vi "cRIO-9076_RT.vi"() -> ()   [LabVIEW 2012]
doc: "This VI shows an example of how to implement a closed loop position move using the NI 9505. The position loop is implemented using PID. The output of the loop is used as the command for the current loop, which then sets the PWM duty cycle for the motor. This example assumes that an encoder is connected for position and velocity feedback. This example does not implement advanced motion features such as trajectory generation and splining."
uses:
  <vilib>/LabVIEW Targets/FPGA/cRIO/cRIO-9505/controls.llb/_nicrio_cRIO-9505_DriveStatus.ctl
  <vilib>/Platform/TimedLoop/XDataNode/timing_clust.ctl
  <vilib>/Platform/TimedLoop/XDataNode/nitl_modes.ctl
  <vilib>/Platform/TimedLoop/XDataNode/wakeup.ctl
  <vilib>/FPGAPlugInAG/cRIO-9076/niLvFpga_Open_cRIO-9076.vi
  <vilib>/Utility/error.llb/Error Cluster From Error Code.vi
  <vilib>/rvi/errors/niLvFpgaAdjustHostInterfaceError.vi
  <vilib>/Analysis/3filter.llb/Zero Phase Filter (DBL).vi
  <vilib>/FPGAPlugInAG/cRIO-9076/niLvFpga_Close_cRIO-9076.vi
  <vilib>/rvi/interface/nirviOpenFPGA/nirviOpenFPGA.xnode
  FPGA Bitfiles/GWiz32_FPGATarget2_PositionControl(_zhcafk1Bo4c.lvbitx
  C:/Temp/National Instruments Downloads/LabVIEW FPGA English/2012SP1/cRIO-9076_FPGA.vi
  <vilib>/rvi/interface/nirviReadWriteControl/nirviReadWriteControl.xnode
  <vilib>/Platform/TimedLoop/XDataNode/XDataNode.xnode
  <vilib>/rvi/interface/nirviCloseFPGA/nirviCloseFPGA.xnode
  NiFpgaLv.dll
  <vilib>/Analysis/NI_AALPro.lvlib
  <vilib>/Platform/TimedLoop/XDataNode/XDNodeRunTimeDep.lvlib
  <vilib>/Analysis/NI_AALBase.lvlib
panel:
  in  "Tab Control":enum32{"Controls", "Plot_data"}(tab)
  in  "samples":i32=10000
  in  "signal type":T1(ring)=enum."square"
  in  "cycles":dbl=1.0 format="%0.2f"
  in  "delay":dbl=180.0 format="%0.2f"
  out "Ball Position (V)":dbl(slide) min=-0.2 max=0.2 step=0.001 scale=0.0..12.0 scale format="%.1f"
  out "Gear Angle Theta (V)":dbl(knob) scale=0.0..12.0 scale format="%.2f"
  in  "MANUAL\n/AUTO":bool caption="Auto"
  in  "Motor Voltage 2":dbl(slide) min=-5.0 max=5.0 step=0.01 scale=-6.0..6.0
  out "Motor Voltage":dbl(knob) scale=-6.0..6.0 scale format="%.1f"
  in  "Stiction V \nOffset cw":dbl step=0.01 format="%.4f"
  in  "dc offset":dbl=0.195 format="%.3f"
  in  "amplitude":dbl=0.075 format="%.3f"
  in  "Period(ms)":dbl=50.0 min=0.1 max=1000.0 format="%.2f"
  out "Period OK":bool=TRUE
  in  "STOP":bool
  out "Missed":i16
  in  "Path":path=path "cRIO-9076_RT.vi"
  in  "Stiction V \nOffset ccw":dbl step=0.01 format="%.4f"
  out "RT Plot":cluster{dbl, "ServoAng":dbl, "BallPosn":dbl}(graph)={0.0, "ServoAng"=7.103515625, "BallPosn"=10.50048828125}
  in  "Data plot":bool
  in  "Ball filter":bool=TRUE
  in  "Gear filter":bool=TRUE
  out "Graph":T2(graph)
  out "error out":errorcluster
  # "GWiz v3.2"
  # "Ball & Beam"
  # "Reference\nGenerator"
  # "F2017 2011"
  # "Press Ctrl-H for help"
  # "Export data: right click plot"
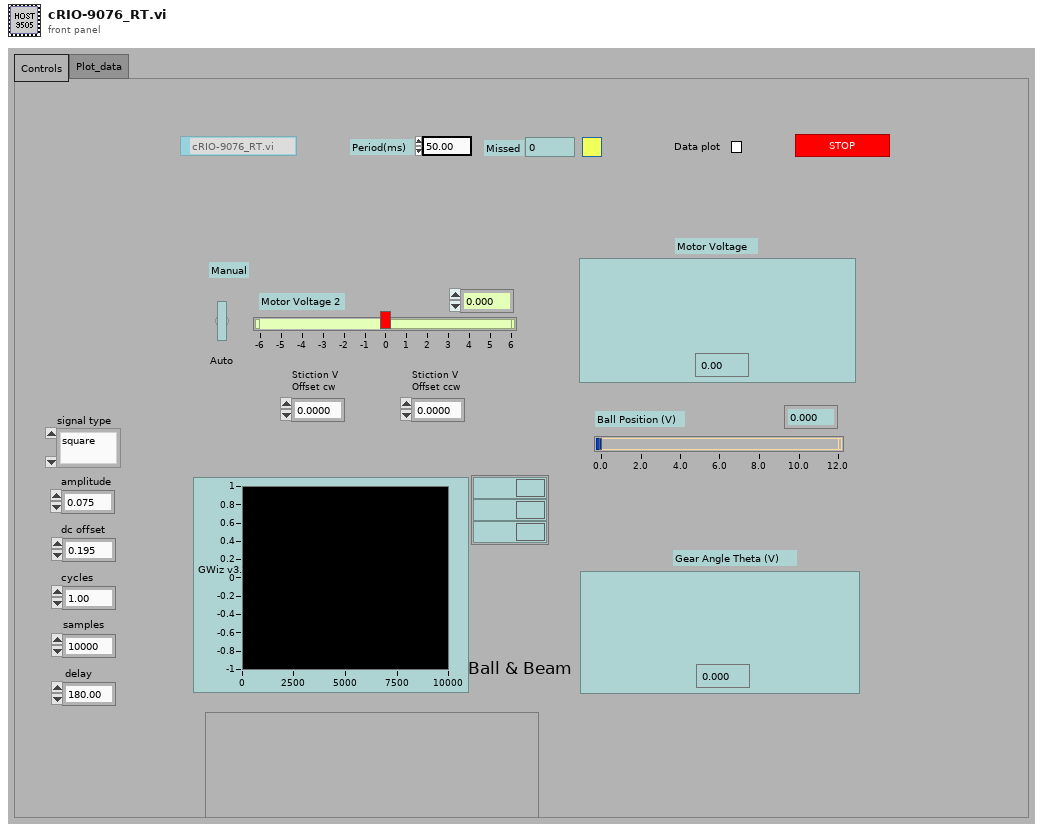
[diagram p1: front panel]
types:
  T1 = enum16{"sine", "cosine", "triangle", "square", "sawtooth", "increasing ramp", "decreasing ramp"}
  T2 = cluster{"Initial time":dbl, dbl, "Data to Plot":dbl[][]}
  T3 = typedef "_nicrio_cRIO-9505_DriveStatus.ctl" = enum8{"Enabled", "Disabled", "Disabled by Drive Fault", "Disabled by Temp. Fault", "Disabled by E-Stop", "Unknown"}
  T4 = typedef "XDNodeRunTimeDep.lvlib/timing_clust.ctl" = cluster{"Expected End [f-1]":u64, "Actual End [f-1]":u64, "Finished Late? [f-1]":bool, "Expected End [i-1]":u64, "Actual End [i-1]":u64, "Finished Late? [i-1]":bool, "Expected Start [i]":u64, "Actual Start [i]":u64, "Expected Start [f]":u64, "Actual Start [f]":u64, "Source Name":string, "Structure Name":string, "Period":i64, "Deadline":i64, "Offset":i64, "Start":i64, "Priority":i32, "Timeout":i32, "Mode":T5, "Wakeup Reason":T6, "Error":errorcluster, "Source Type":string, "Secondary Source Type":string, "Global End Time":u64, "Global Start Time":u64, "Frame Duration":u64, "Iteration Duration":u64, "Assigned CPU":i32, "I/O Scan Engine Mode":u32}
  T5 = typedef "XDNodeRunTimeDep.lvlib/nitl_modes.ctl" = enum32{"No Change", "Process missed periods, maintain original phase", "Discard missed periods, maintain original phase", "Process missed periods, ignore original phase", "Discard missed periods, ignore original phase"}
  T6 = typedef "XDNodeRunTimeDep.lvlib/wakeup.ctl" = enum32{"Normal", "Aborted", "Asynchronous wakeup", "Timing source error", "Timed loop error", "Timeout"}
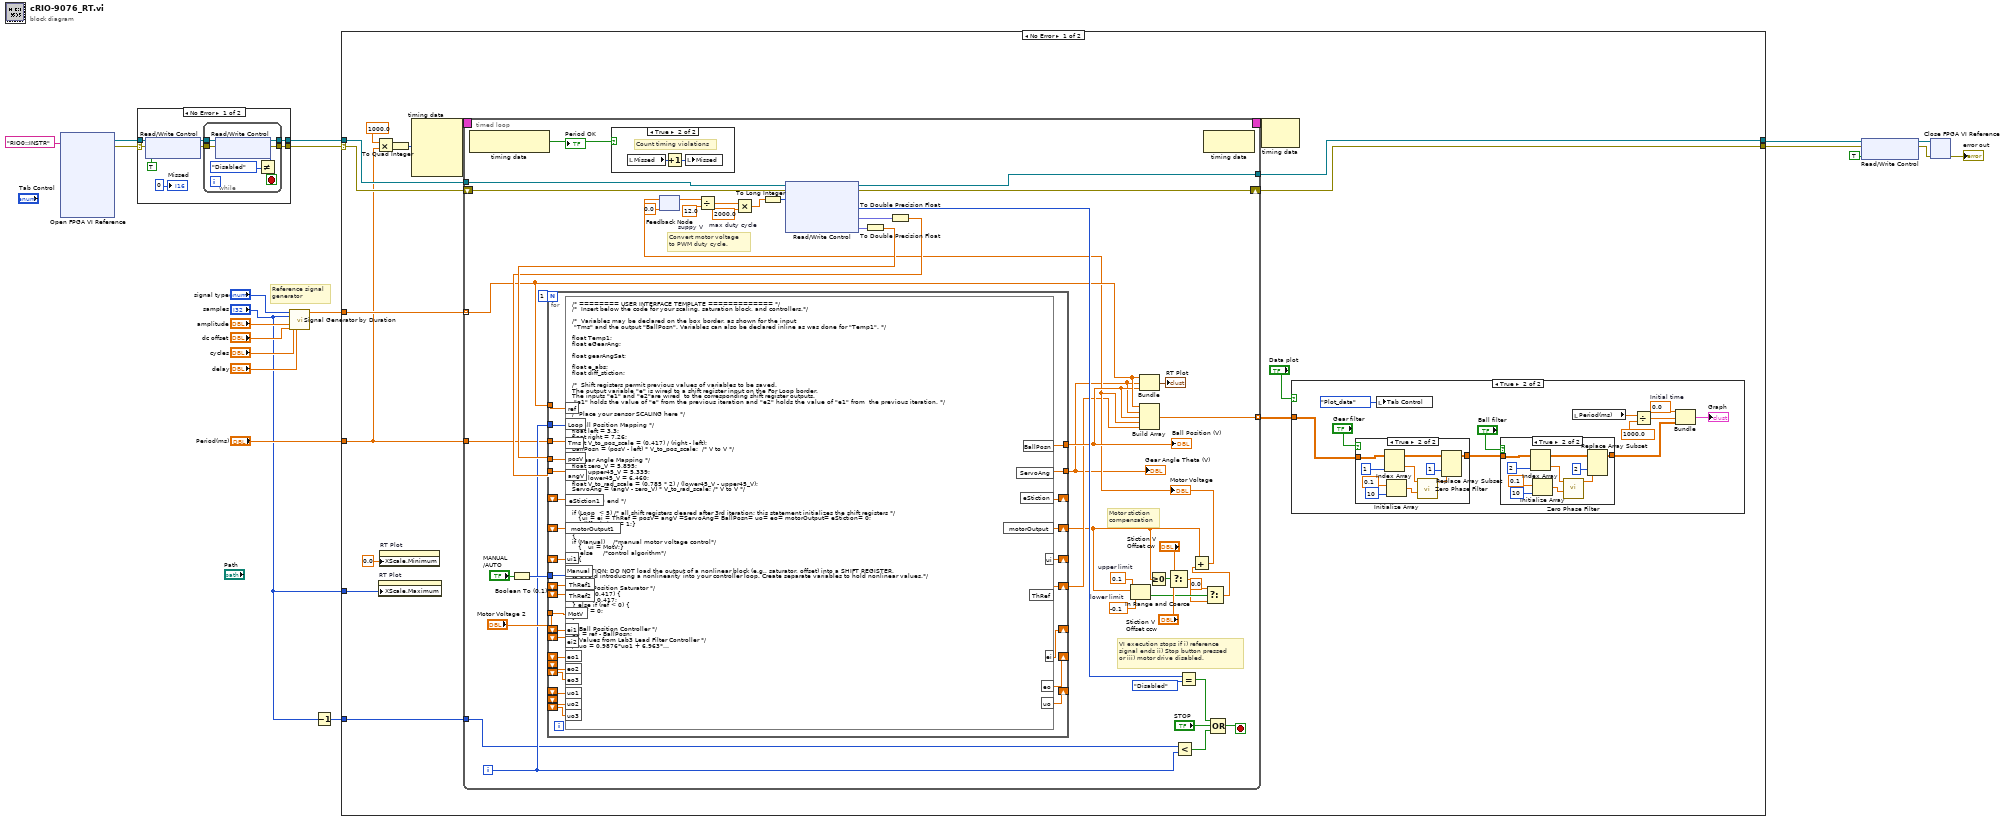
[diagram p0: block diagram]
diagram:
  # "Reference signal\ngenerator"
  n1 = xnode "Open FPGA VI Reference"("resource name"="RIO0::INSTR") -> ("FPGA VI Reference Out"=w7:refnum<k20>, "error out"=w14:errorcluster)  [unwired: 1 in]
  n2 = case shown="No Error" w14 {
    selector: w14 -> [w23 w36]
    tunnel: w7 -> [w26 w37]
    tunnel: [w28 w37] -> w15
    tunnel: [w22 w36] -> w13
    frame No Error {
      n3 = xnode "Read/Write Control"("FPGA VI Reference In"=w26, "error in"=w23, "Enable Drive"=TRUE) -> ("FPGA VI Reference Out"=w25:refnum<k20>, "error out"=w24:errorcluster)
      n4 = while {
        tunnel: [w35] -> w28
        tunnel: w25 -> [w31]
        tunnel: w24 -> [w32]
        tunnel: [w29] -> w22
        stop <- w30 stop-if-true
        n5 = xnode "Read/Write Control"("FPGA VI Reference In"=w31, "error in"=w32) -> ("FPGA VI Reference Out"=w35:refnum<k20>, "error out"=w29:errorcluster, "Drive Status"=w34:T3)
        n6 = Not Equal?(x=w34, y=_nicrio_cRIO-9505_DriveStatus."Disabled") -> (x != y?=w30:bool)
      }
      "Missed" <- i16 0 ("Missed")
    }
    frame Error {
      # "Error occurred. Do not run."
    }
  }
  n7 = call <vilib>:"Signal Generator by Duration.vi"("signal type"="signal type", "# of samples"="samples", "frequency"="cycles", "amplitude"="amplitude", "dc offset"="dc offset", "phase in"="delay") -> ("signal"=w9:dbl[])  [unwired: 6 in, 3 out]
  n8 = Decrement(x="samples") -> (x-1=w2:i32)
  n9 = case shown="No Error" w13 {
    selector: w13 -> [w51 w169]
    tunnel: w15 -> [w53 w170]
    tunnel: [w42 w170] -> w20
    tunnel: [w52 w169] -> w19
    tunnel: w9 -> [w50 _]
    tunnel: w2 -> [w49 _]
    tunnel: "Period(ms)" -> [w46 _]
    tunnel: "samples" -> [w38 _]
    frame No Error {
      n10 = Multiply(x=1000.0, y=w46) -> (x*y=w44:dbl)
      n11 = property on="RT Plot" class="WFChart (strict)"("XScale.Maximum"=w38) -> ()  [unwired: 2 in, 2 out]
      n12 = property on="RT Plot" class="WFChart (strict)"("XScale.Minimum"=0.0 ("X Scale.Range:Minimum")) -> ()  [unwired: 2 in, 2 out]
      n13 = To Quad Integer(1:w44) -> (0:w43:i64)
      n14 = node-c288(w43) -> (w48:T4)  [unwired: 3 in]
      n15 = timed-loop {
        tunnel: w53 -> [w130]
        tunnel: [w128] -> w42
        shift-right: [w127] -> w52
        shift-left: w51 -> [w129]
        tunnel: w50 -> [w101] mode=indexing
        tunnel: w49 -> [w103]
        tunnel: w46 -> [w96]
        timing: w48 -> [_]
        timing-out: [_] -> w47
        tunnel: [w97] -> w41 mode=indexing
        i -> [w104]
        stop <- w124 stop-if-true
        w89 = -0.1  # lower limit
        w90 = 0.1  # upper limit
        w109 = 2000.0  # max duty cycle
        w108 = 12.0  # suppy V
        # "Convert motor voltage\nto PWM duty cycle."
        # "VI execution stops if i) reference\nsignal ends ii) Stop button pressed\nor iii) motor drive disabled."
        # "Motor stiction\ncompensation"
        n16 = node-c288() -> (w111:bool)  [unwired: 1 in]
        "Period OK" <- w111
        n17 = Boolean To (0,1)(Boolean="MANUAL\n/AUTO") -> (0, 1=w116:i16)
        n18 = case shown="True" w111 {
          frame False {
          }
          frame True {
            # "Count timing violations"
            n19 = local read "Missed"() -> (w132:i16)
            n20 = Increment(x=w132) -> (x+1=w131:i16)
            n21 = local write "Missed"(w131) -> ()
          }
        }
        n22 = feedback #1(0.0) -> (w106:dbl)
        n23 = Divide(x=w106, y=w108) -> (x/y=w107:dbl)
        n24 = Multiply(x=w107, y=w109) -> (x*y=w105:dbl)
        n25 = To Long Integer(number=w105) -> (32bit integer=w102:i32)
        n26 = xnode "Read/Write Control"("FPGA VI Reference In"=w130, "error in"=w129, "Position Setpoint"=w102) -> ("FPGA VI Reference Out"=w128:refnum<k20>, "error out"=w127:errorcluster, "Drive Status"=w126:T3, "Gear Pot"=w122:fxp<+/-,16,5>, "Ball Pot"=w121:fxp<+/-,16,5>)
        n27 = To Double Precision Float(number=w121) -> (double precision float=w119:dbl)
        n28 = To Double Precision Float(number=w122) -> (double precision float=w114:dbl)
        n29 = for {
          N: 1 -> [_]
          tunnel: w101 -> [w164]
          tunnel: w119 -> [w163]
          shift-right: [w149] -> w88
          shift-left: _ -> [w162]
          shift-right: [w161] -> _
          shift-left: _ -> [w160]
          tunnel: [w159] -> w100
          tunnel: w96 -> [w158]
          tunnel: w114 -> [w157]
          tunnel: [w156] -> w95
          tunnel: w116 -> [w155]
          tunnel: "Motor Voltage 2" -> [w154]
          shift-right: [w153] -> w98
          shift-left: _ -> [w152]
          shift-left: _ -> [w151]
          tunnel: w104 -> [w150]
          shift-left: _ -> [w148]
          shift-right: [w146] -> _
          shift-left: _ -> [w147]
          shift-left: _ -> [w145]
          shift-right: [w144] -> _
          shift-left: _ -> [w143]
          shift-left: _ -> [w142]
          shift-right: [w141] -> _
          shift-left: _ -> [w140]
          shift-right: [w139] -> _
          shift-left: _ -> [w138]
          shift-left: _ -> [w137]
          shift-left: _ -> [w136]
          n30 = formula code="/* ======== USER INTERFACE TEMPLATE ============= */\n/*  Insert below the code for your scaling, saturation block, and controllers.*/\n\n/*  Variables may be declared on the box border, as shown for the input \n \"Tms\" and the output \"BallPosn\". Variables can also be declared inline as was done for \"Temp1\". */\n\nfloat Temp1; \nfloat eGearAng;\n\nfloat gearAngSat;\n\nfloat e_abs;\nfloat diff_stiction;\n\n/*  Shift registers permit previous values of variables to be saved. \nThe output variable \"e\" is wired to a shift register input on the For Loop border.  \nThe inputs \"e1\" and \"e2\"are wired  to the corresponding shift register outputs.\n \"e1\" holds the value of \"e\" from the previous iteration and \"e2\" holds the value of \"e1\" from  the previous iteration. */\n\n/* Place your sensor SCALING here */\n\n/* Ball Position Mapping */\nfloat left = 3.3;\nfloat right = 7.26;\nfloat V_to_pos_scale = (0.417) / (right - left);\nBallPosn = (posV - left) * V_to_pos_scale;  /* V to V */\n\n/* Gear Angle Mapping */\nfloat zero_V = 5.895;\nfloat upper45_V = 5.339;\nfloat lower45_V = 6.460;\nfloat V_to_rad_scale = (0.785 * 2) / (lower45_V - upper45_V);\nServoAng = (angV - zero_V) * V_to_rad_scale; /* V to V */\n\n/* SCALING end */\n\nif (Loop  < 5) /* all shift registers cleared after 3rd iteration; this statement initializes the shift registers */\n   {ui = ei = ThRef = posV= angV =ServoAng= BallPosn= uo= eo= motorOutput= eStiction= 0;\n     diff_stiction = 1;}\nelse\n{\nif (Manual)    /*manual motor voltage control*/\n   {   ui = MotV;}\n    else     /*control algorithm*/\n   { \n\n/* CAUTION: DO NOT load the output of a nonlinear block (e.g., saturator, offset) into a SHIFT REGISTER, \nto avoid introducing a nonlinearity into your controller loop. Create separate variables to hold nonlinear values.*/\n\n/* Ball Position Saturator */\nif(ref > 0.417) {\n    ref = 0.417;\n} else if (ref < 0) {\n    ref = 0;\n}\n\n/* Ball Position Controller */\neo = ref - BallPosn;\n/* Values from Lab3 Lead Filter Controller */\n/* uo = 0.9876*uo1 + 6.963*eo - 6.95*eo1; */\n\n/* Values from Lab3 Pole Placement Controller */\nuo =  9.947828571*eo - 19.87577143*eo1 + 9.927952795*eo2 + 1.98757764*uo1 - 0.9875776398*uo2;\nThRef = gearAngSat = uo;\n\ne_abs = eo;\nif(e_abs < 0) {e_abs = -1*e_abs;}\nif(Loop % 10 == 0) {\n    eStiction = e_abs;\n    diff_stiction = eStiction - eStiction1;\n}\nif(e_abs < 0.05 && e_abs > 0.005 && diff_stiction < 0.01){\n        /*if(eo > 0){\n            gearAngSat = gearAngSat + 0.2;\n        }\n        if(eo < 0){\n            gearAngSat = gearAngSat - 0.2;\n        }*/\n        gearAngSat = gearAngSat + eo*4;\n    }\n\n/* Gear Angle Saturator */\nif(gearAngSat  > 0.785) {\n    gearAngSat  = 0.785;\n} else if (gearAngSat  < -0.785) {\n    gearAngSat  = -0.785;\n}\n\n/* Gear Aangle Controller */\n  ei = gearAngSat - ServoAng;\n  ui = 0.9488*ui1 + 14.98*ei - 14.25*ei1; /* Values from Lab2.m */\n  motorOutput = ui;\n\n\n/* Motor Power Saturator */\n  if(motorOutput>6) {\n    motorOutput=6;\n  } else if(motorOutput<-6) {\n    motorOutput=-6;\n  }\n\n   }\n} \n    \n/* ThRef, ThRef1, e, e1 are present, but not used in this demo.  \nHowever, they will be necessary (at a minimum) when the controllers will be implemented. */"("Tms"=w158, "Loop"=w150, "motorOutput1"=w162, "ei1"=w160, "ref"=w164, "posV"=w163, "angV"=w157, "Manual"=w155, "MotV"=w154, "ThRef1"=w152, "ei2"=w151, "ThRef2"=w148, "eo1"=w147, "eo2"=w145, "uo1"=w143, "uo2"=w142, "eStiction1"=w140, "ui1"=w138, "uo3"=w137, "eo3"=w136) -> ("motorOutput"=w149:dbl, "ei"=w161:dbl, "BallPosn"=w159:dbl, "ServoAng"=w156:dbl, "ThRef"=w153:dbl, "eo"=w146:dbl, "uo"=w144:dbl, "eStiction"=w141:dbl, "ui"=w139:dbl)
        }
        "Ball Position (V)" <- w100
        "Gear Angle Theta (V)" <- w95
        n31 = In Range and Coerce(upper limit=w90, x=w88, lower limit=w89) -> (In Range?=w87:bool)  [unwired: 1 out]
        n32 = Bundle(w101, "ServoAng"=w95, "BallPosn"=w100) -> (→"RT Plot":cluster{dbl, "ServoAng":dbl, "BallPosn":dbl})  [unwired: 1 in]
        n33 = Greater Or Equal To 0?(x=w88) -> (x >= 0?=w113:bool)
        n34 = Select(t="Stiction V \nOffset cw", s=w113, f="Stiction V \nOffset ccw") -> (s? t:f=w86:dbl)
        n35 = Less?(x=w103, y=w104) -> (x < y?=w115:bool)
        n36 = Equal?(x=w126, y=_nicrio_cRIO-9505_DriveStatus."Disabled") -> (x = y?=w123:bool)
        n37 = node-c288() -> ()  [unwired: 1 in, 1 out]
        n38 = Select(t=0.0, s=w87, f=w86) -> (s? t:f=w93:dbl)
        n39 = Add(x=w88, y=w93) -> (x+y=w99:dbl)
        "Motor Voltage" <- w99
        n40 = feedback-in #1(w99) -> ()
        n41 = Build Array(w101, w95, w100, w99, w98) -> (w97:dbl[])
        n42 = Compound Arithmetic op=OR(w123, "STOP", w115) -> (w124:bool)
      }
      n43 = node-c288(w47) -> ()  [unwired: 1 out]
      n44 = case shown="True" "Data plot" {
        tunnel: w41 -> [_ w59]
        frame False {
        }
        frame True {
          w64 = 0.0  # Initial time
          n45 = case shown="True" "Gear filter" {
            tunnel: w59 -> [w75 w77]
            tunnel: [w75 w76] -> w61
            frame False {
            }
            frame True {
              n46 = Index Array(array=w77, index (col)=1 ("index (row)")) -> (element=w79:dbl[])  [unwired: 1 in]
              n47 = Initialize Array(0.1 ("element"), 10 ("dimension size")) -> (w82:dbl[])
              n48 = call-poly <vilib>:"Zero Phase Filter.vi"("Forward Coefficients"=w82, "X"=w79) -> ("Filtered X"=w78:dbl[])  [unwired: 8 in, 1 out]
              n49 = Replace Array Subset(array=w77, new element=w78, index (col)=1 ("disabled index (col)")) -> (w76:dbl[][])  [unwired: 1 in]
            }
          }
          n50 = local write "Tab Control"(enum32{"Controls", "Plot_data"}."Plot_data" ("Tab Control")) -> ()
          n51 = case shown="True" "Ball filter" {
            tunnel: w61 -> [w65 w67]
            tunnel: [w65 w66] -> w60
            frame False {
            }
            frame True {
              n52 = Index Array(array=w67, index (col)=2 ("index (row)")) -> (element=w69:dbl[])  [unwired: 1 in]
              n53 = Initialize Array(0.1 ("element"), 10 ("dimension size")) -> (w72:dbl[])
              n54 = call-poly <vilib>:"Zero Phase Filter.vi"("Forward Coefficients"=w72, "X"=w69) -> ("Filtered X"=w68:dbl[])  [unwired: 8 in, 1 out]
              n55 = Replace Array Subset(array=w67, new element=w68, index (col)=2 ("disabled index (col)")) -> (w66:dbl[][])  [unwired: 1 in]
            }
          }
          n56 = local read "Period(ms)"() -> (w58:dbl)
          n57 = Divide(x=w58, y=1000.0) -> (x/y=w62:dbl)
          n58 = Bundle("Initial time"=w64, w62, w60) -> (→"Graph":cluster{"Initial time":dbl, dbl, dbl[][]})  [unwired: 1 in]
        }
      }
    }
    frame Error {
      # "Error occurred. Do not run."
    }
  }
  n59 = xnode "Read/Write Control"("FPGA VI Reference In"=w20, "error in"=w19, "Disable Drive"=TRUE) -> ("FPGA VI Reference Out"=w18:refnum<k20>, "error out"=w17:errorcluster)
  n60 = xnode "Close FPGA VI Reference"("FPGA VI Reference In"=w18, "error in"=w17) -> ("error out"=→"error out":errorcluster)
